vi "bats.parser.vi"(10 "niInstr IPv4 UDP Data Stream out":refnum<class "niInstr IPv4 UDP Data Stream v1.lvclass">, 11 "reset":bool) -> (2 "Ready.for.Udp.Input":bool)   [LabVIEW 2020]
uses:
  <instrlib>/_niInstr/Network/IPv4/UDP/Data Stream/v1/niInstr IPv4 UDP Data Stream v1.lvclass
  bats.parser.state.data.ctl
  bats.parser.state.command.ctl
  debug/debug.type.ctl
  <instrlib>/_niInstr/Network/IPv4/UDP/Data Stream/v1/Read Data Stream.vi
  <vilib>/rvi/Emulation/niFpgaEmulationIsFPGAContextNoSignature.vi
  <vilib>/rvi/Emulation/niFpgaSctlEmulationGetInTimedLoop.vi
  <vilib>/rvi/errors/niFpgaSetErrorForExecOnDevCompSimple.vi
  <vilib>/rvi/eio/common/nirviEmuReportErrorAndStop.vi
  <vilib>/rvi/DataTransferAndStorage/Container/Common/niFpgaContainerGetUniqueNameForEmu.vi
  <vilib>/rvi/FIFO/Fifo_Resource/nirvififoEmulationSetSize.vi
  <vilib>/rvi/FIFO/Fifo_Resource/nirviFifoEmulationQueueMgr.vi
  <instcachedir>/0/nirviFifoEmulationQueueMgr_E5CAEC123FF24DC58D834DCA3CDAA9B5.lvgen/nirviFifoEmulationQueueMgr_E5CAEC123FF24DC58D834DCA3CDAA9B5_008.vi
  <vilib>/rvi/FIFO/Fifo_Resource/nirvififoEmulationDetermineInputValidOut.vi
  <vilib>/rvi/FIFO/Fifo_Resource/nirvififoEmulationCreateLock.vi
  <vilib>/rvi/Emulation/niFpgaProcessEmulError.vi
  <vilib>/rvi/FIFO/Fifo_Resource/nirvififoEmulationObtainLock.vi
  <vilib>/rvi/FIFO/Fifo_Resource/nirvififoEmulationReleaseLock.vi
  <vilib>/rvi/occurrence/nirviWaitOnOccurrenceBase.vi
  <vilib>/rvi/errors/nirviReportUnexpectedCaseInternalError.vi
  <vilib>/rvi/errors/nirviReportUnexpectedCaseInternalError (U32).vi
  <instcachedir>/0/nirviFifoEmulationQueueMgr_E5CAEC123FF24DC58D834DCA3CDAA9B5.lvgen/nirviFifoEmulationQueueMgr_E5CAEC123FF24DC58D834DCA3CDAA9B5_006.vi
  <vilib>/rvi/DataTransferAndStorage/Container/XNode/niFpgaContainer.xnode
  <vilib>/rvi/FIFO/Fifo_Resource/nirvififoEmulationWrite.vi
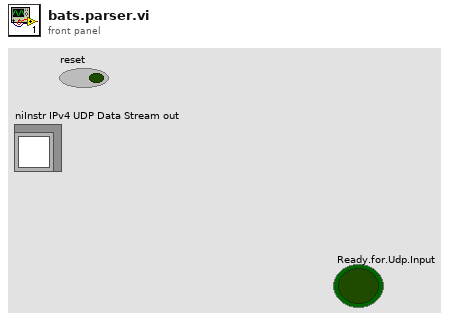
[diagram p1: front panel]
types:
  T1 = typedef "bats.parser.state.command.ctl" = enum16{"Reset", "Noop", "Read.Sequenced.Unit.Header", "Read.Msg"}
  T2 = typedef "bats.parser.state.data.ctl" = cluster{"BATS.Parser.States":T1, "Saved.BATS.Parser.State":T1, "Hdr Length (U16)":u16, "MessageLength (U8)":u8, "MessageType (U8)":u8, "Time (U32)":u32, "Total Counter (U16)":u16, "Message Counter (U8)":u8, "i":u16, "Number.of.Tickers":u16, "n":u16, "msg.counter":u8, "msg.length":u8, "buffer.start":u8, "buffer.length":u8, "buffer":u64[], "Debug":T3, "Next.Seq.No":u32}
  T3 = typedef "debug.type.ctl" = cluster{"Write.to.Debug":bool, "Data":u64}
  T4 = typedef "niInstr Ethernet Utilities FPGA v1.lvlib/Network Data Stream.ctl" = cluster{"data":u8[], "data valid":bool, "byte enables":bool[]}
  T5 = typedef "fpganow.common.fpga.lvlib/orderbook.command.ctl" = cluster{"type":T6, "side":u8, "orderId ":u64, "quantity":u32, "symbol":u64, "price":u64, "executed.qty":u32, "canceled.qty":u32, "remaining.qty":u32, "seconds":u64, "nanoseconds":u64, "Add":bool, "Edit":bool, "Remove":bool, "seq no":u32}
  T6 = typedef "fpganow.common.fpga.lvlib/orderbook.command.type.ctl" = enum8{"Time", "AddOrder", "OrderExecuted", "OrderExecutedAtPrice", "ReduceSize", "ModifyOrder", "DeleteOrder", "Get.Everything", "Get.All.Orders", "Get.Top"}
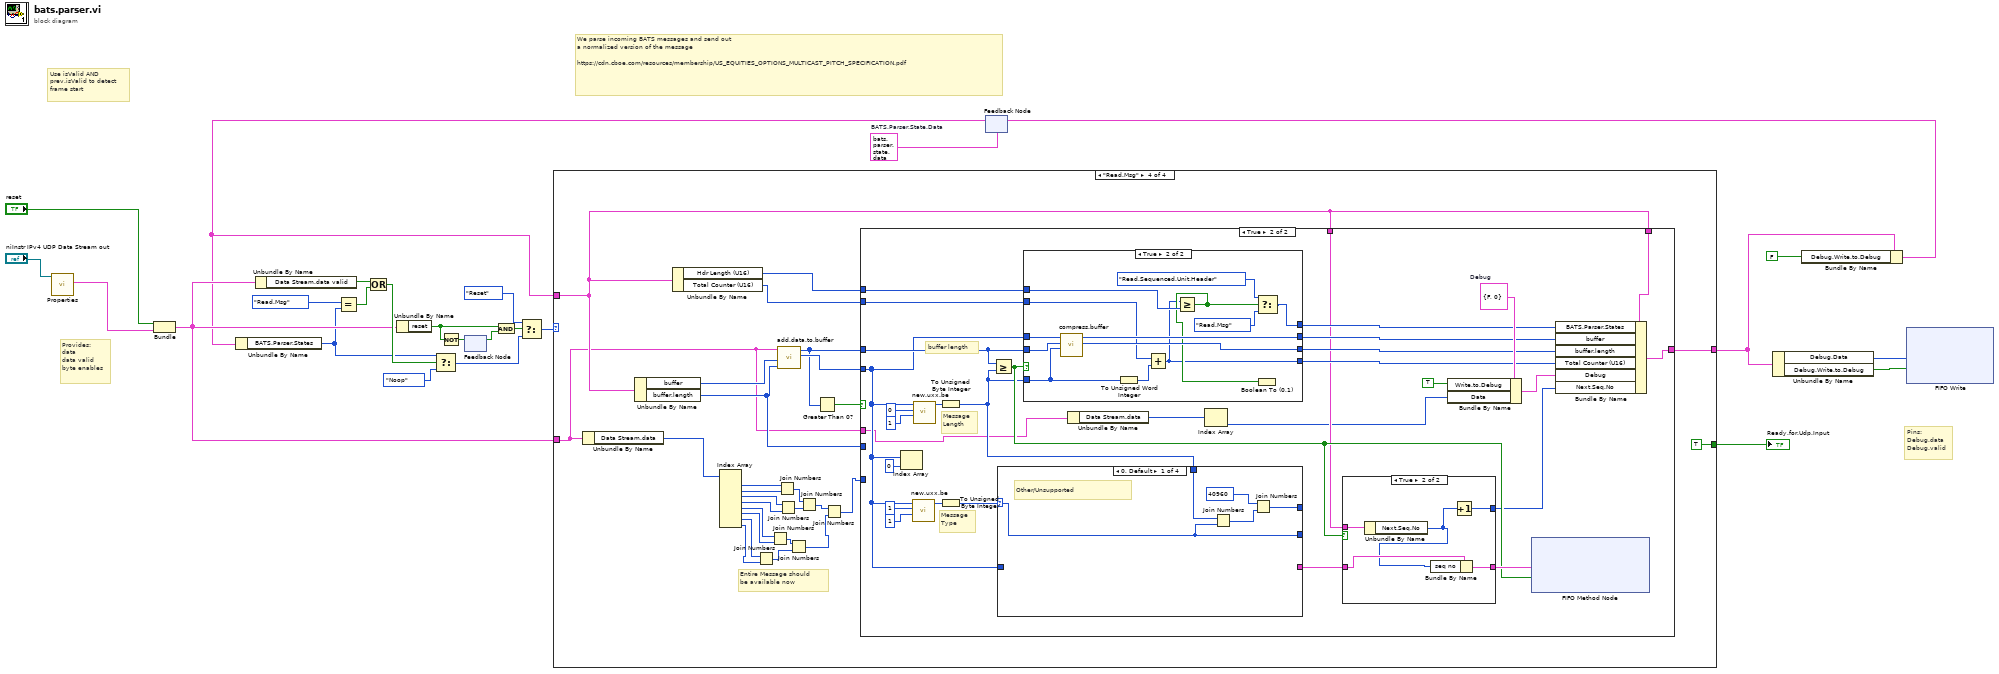
[diagram p0: block diagram]
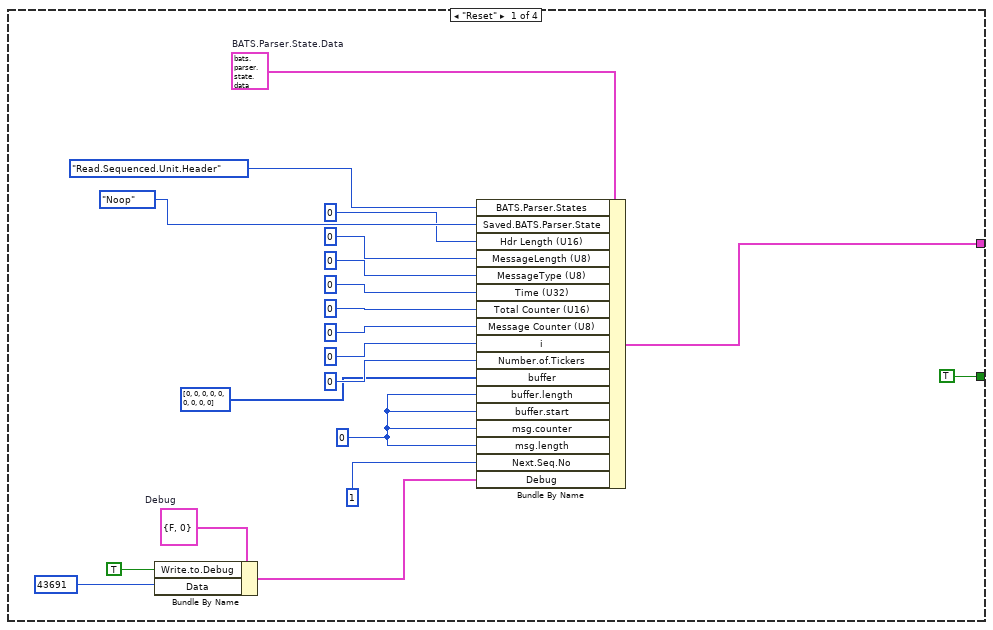
[diagram p2: hidden frame]
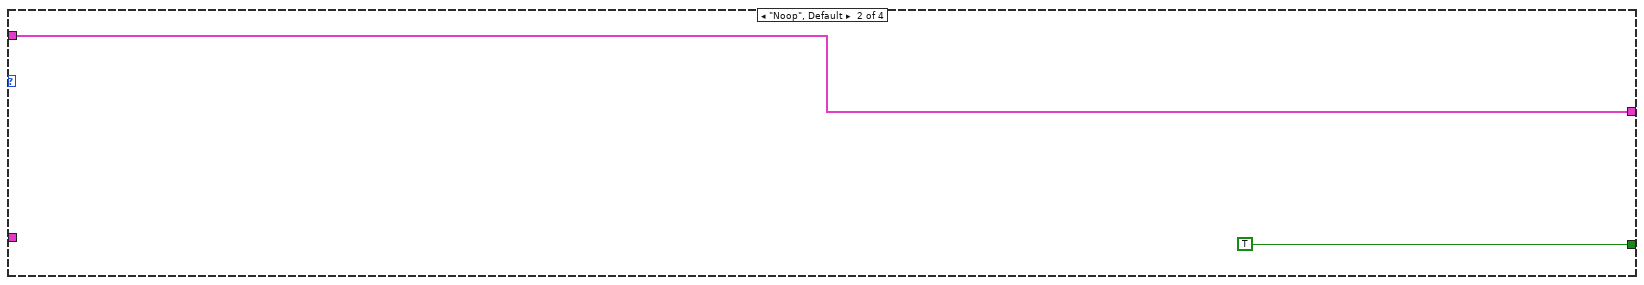
[diagram p3: hidden frame]
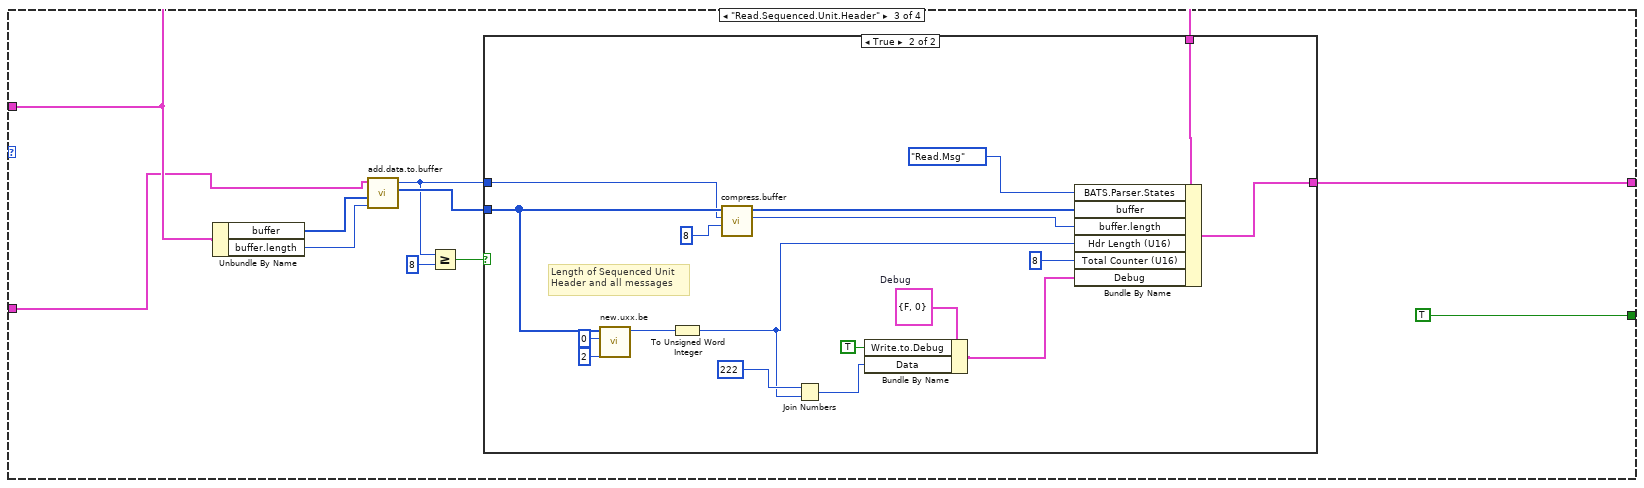
[diagram p4: hidden frame]
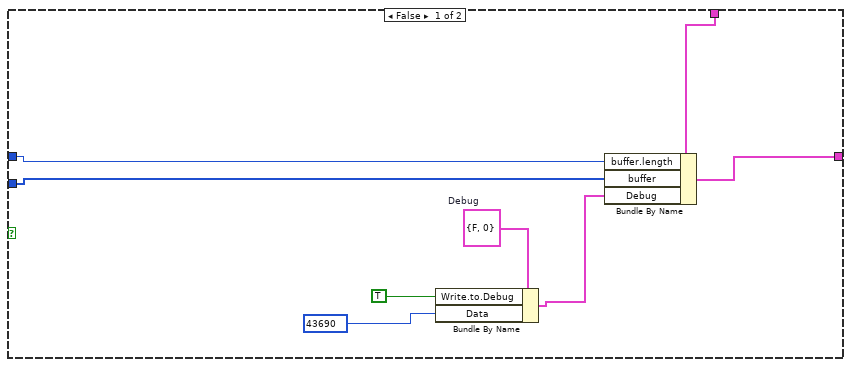
[diagram p5: hidden frame]
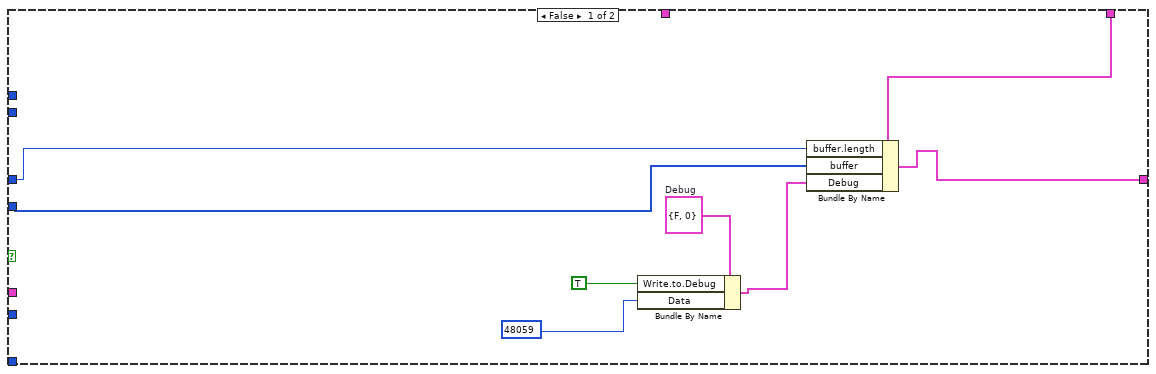
[diagram p6: hidden frame]
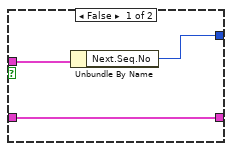
[diagram p7: hidden frame]
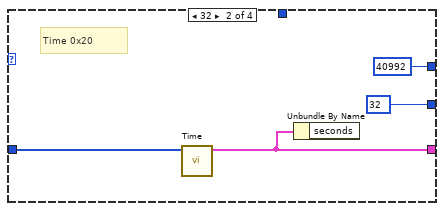
[diagram p8: hidden frame]
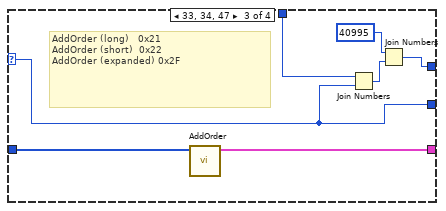
[diagram p9: hidden frame]
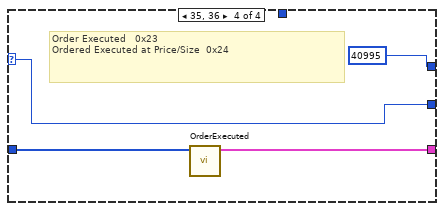
[diagram p10: hidden frame]
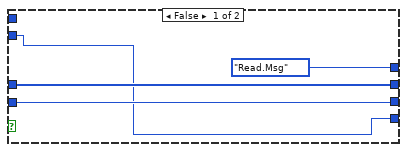
[diagram p11: hidden frame]
diagram:
  w25 = T2 {"BATS.Parser.States"=enum."Read.Sequenced.Unit.Header", "Saved.BATS.Parser.State"=enum."Reset", "Hdr Length (U16)"=0, "MessageLength (U8)"=0, "MessageType (U8)"=0, "Time (U32)"=0, "Total Counter (U16)"=0, "Message Counter (U8)"=0, "i"=0, "Number.of.Tickers"=0, "n"=0, "msg.counter"=0, "msg.length"=0, "buffer.start"=0, "buffer.length"=0, "buffer"=[0, 0, 0, 0, 0, 0, 0, 0, 0], "Debug"={"Write.to.Debug"=FALSE, "Data"=0}, "Next.Seq.No"=0}  # BATS.Parser.State.Data
  # "Use isValid AND\nprev.isValid to detect\nframe start"
  # "Provides:\ndata\ndata valid\nbyte enables"
  # "Pins:\nDebug.data\nDebug.valid"
  # "We parse incoming BATS messages and send out\na normalized version of the message\n\nhttps://cdn.cboe.com/resources/membership/US_EQUITIES_OPTIONS_MULTICAST_PITCH_SPECIFICATION.pdf"
  n1 = call-poly <instrlib>:"Properties.vi"("niInstr IPv4 UDP Data Stream v1.lvclass"="niInstr IPv4 UDP Data Stream out") -> ("Data Stream"=w2:T4)  [unwired: 9 in, 1 out]
  n2 = Bundle("reset"="reset", "Data Stream"=w2) -> (w9:cluster{"reset":bool, "Data Stream":T4})  [unwired: 1 in]
  n3 = Unbundle By Name(w9) -> ("Data Stream.data valid"=w12:bool)
  n4 = Unbundle By Name(w9) -> ("reset"=w15:bool)
  n5 = Not(x=w15) -> (.not. x?=w17:bool)
  n6 = feedback-in #1(w17) -> ()
  n7 = feedback #1() -> (w18:bool)  [unwired: 1 in]
  n8 = And(x=w15, y=w18) -> (x .and. y?=w19:bool)
  n9 = feedback #2(w25) -> (w1:T2)
  n10 = Unbundle By Name(w1) -> ("BATS.Parser.States"=w8:T1)
  n11 = Equal?(x=bats.parser.state.command."Read.Msg" ("BATS.Parser.States"), y=w8) -> (x = y?=w20:bool)
  n12 = Compound Arithmetic op=OR(w12, w20) -> (w11:bool)
  n13 = Select(t=w8, s=w11, f=bats.parser.state.command."Noop" ("BATS.Parser.States")) -> (s? t:f=w10:T1)
  n14 = Select(t=bats.parser.state.command."Reset" ("BATS.Parser.States"), s=w19, f=w10) -> (s? t:f=w22:T1)
  n15 = case shown="\"Read.Msg\"" w22 {
    tunnel: w1 -> [_ w47 w53 w102]
    tunnel: [w44 w47 w55 w110] -> w4
    tunnel: [TRUE ("Ready for Input") TRUE ("Ready for Input") TRUE ("Ready for Input") TRUE ("Ready for Input")] -> w16
    tunnel: w9 -> [_ _ w48 w84]
    frame "Reset" {
      w33 = T3 {"Write.to.Debug"=FALSE, "Data"=0}  # Debug
      w27 = u8 0 ("buffer.length")
      w45 = T2 {"BATS.Parser.States"=enum."Read.Sequenced.Unit.Header", "Saved.BATS.Parser.State"=enum."Reset", "Hdr Length (U16)"=0, "MessageLength (U8)"=0, "MessageType (U8)"=0, "Time (U32)"=0, "Total Counter (U16)"=0, "Message Counter (U8)"=0, "i"=0, "Number.of.Tickers"=0, "n"=0, "msg.counter"=0, "msg.length"=0, "buffer.start"=0, "buffer.length"=0, "buffer"=[0, 0, 0, 0, 0, 0, 0, 0, 0], "Debug"={"Write.to.Debug"=FALSE, "Data"=0}, "Next.Seq.No"=0}  # BATS.Parser.State.Data
      n16 = Bundle By Name(cluster=w33, "Write.to.Debug"=TRUE, "Data"=u64 43691) -> (w28:T3)
      n17 = Bundle By Name(cluster=w45, "BATS.Parser.States"=bats.parser.state.command."Read.Sequenced.Unit.Header", "Saved.BATS.Parser.State"=bats.parser.state.command."Noop" ("BATS.Parser.States"), "Hdr Length (U16)"=u16 0, "MessageLength (U8)"=u8 0, "MessageType (U8)"=u8 0, "Time (U32)"=u32 0, "Total Counter (U16)"=u16 0, "Message Counter (U8)"=u8 0, "i"=u16 0, "Number.of.Tickers"=u16 0, "buffer"=u64[] [0, 0, 0, 0, 0, 0, 0, 0, 0], "buffer.length"=w27, "buffer.start"=w27, "msg.counter"=w27, "msg.length"=w27, "Next.Seq.No"=u32 1, "Debug"=w28) -> (w44:T2)
    }
    frame "Noop", Default {
    }
    frame "Read.Sequenced.Unit.Header" {
      n18 = Unbundle By Name(w53) -> ("buffer"=w57:u64[], "buffer.length"=w56:u8)
      n19 = call "add.data.to.buffer.vi"("buffer.length"=w56, "buffer"=w57, "network Data Stream.ctl"=w48) -> ("buffer.out"=w54:u64[], "buffer.length.out"=w51:u8)  [unwired: 7 in]
      n20 = Greater Or Equal?(x=w51, y=u8 8) -> (x >= y?=w52:bool)
      n21 = case shown="True" w52 {
        tunnel: [w62 w83] -> w55
        tunnel: w54 -> [w59 w78]
        tunnel: w51 -> [w60 w70]
        tunnel: w53 -> [w61 w81]
        frame False {
          w63 = T3 {"Write.to.Debug"=FALSE, "Data"=0}  # Debug
          n22 = Bundle By Name(cluster=w63, "Write.to.Debug"=TRUE, "Data"=u64 43690) -> (w65:T3)
          n23 = Bundle By Name(cluster=w61, "buffer.length"=w60, "buffer"=w59, "Debug"=w65) -> (w62:T2)
        }
        frame True {
          w74 = T3 {"Write.to.Debug"=FALSE, "Data"=0}  # Debug
          # "Length of Sequenced Unit\nHeader and all messages"
          n24 = call "new.uxx.be.vi"("buffer (U64)"=w78, "Start.Idx"=u8 0, "Length"=u8 2) -> ("Uxx.be"=w75:u64)  [unwired: 7 in]
          n25 = To Unsigned Word Integer(number=w75) -> (unsigned 16bit integer=w66:u16)
          n26 = call "compress.buffer.vi"("start.idx"=u8 8, "buffer.length"=w70, "buffer"=w78) -> ("buffer.length.out"=w69:u8, "buffer.out"=w76:u64[])  [unwired: 7 in]
          n27 = Join Numbers(hi=u32 222 ("Data"), lo=w66) -> ((hi.lo)=w67:u64)
          n28 = Bundle By Name(cluster=w74, "Write.to.Debug"=TRUE, "Data"=w67) -> (w72:T3)
          n29 = Bundle By Name(cluster=w81, "BATS.Parser.States"=bats.parser.state.command."Read.Msg", "buffer"=w76, "buffer.length"=w69, "Hdr Length (U16)"=w66, "Total Counter (U16)"=u16 8, "Debug"=w72) -> (w83:T2)
        }
      }
    }
    frame "Read.Msg" {
      # "Entire Message should \nbe available now"
      n30 = Unbundle By Name(w84) -> ("Data Stream.data"=w85:u8[])
      n31 = Unbundle By Name(w102) -> ("buffer"=w101:u64[], "buffer.length"=w104:u8)
      n32 = Unbundle By Name(w102) -> ("Hdr Length (U16)"=w106:u16, "Total Counter (U16)"=w105:u16)
      n33 = Index Array(array=w85) -> (element #1=w100:u8, element #2=w99:u8, element #3=w98:u8, element #4=w97:u8, element #5=w96:u8, element #6=w95:u8, element #7=w94:u8, element #8=w93:u8)  [unwired: 8 in]
      n34 = Join Numbers(hi=w94, lo=w93) -> ((hi.lo)=w92:u16)
      n35 = Join Numbers(hi=w96, lo=w95) -> ((hi.lo)=w91:u16)
      n36 = Join Numbers(hi=w100, lo=w99) -> ((hi.lo)=w89:u16)
      n37 = Join Numbers(hi=w98, lo=w97) -> ((hi.lo)=w90:u16)
      n38 = call "add.data.to.buffer.vi"("buffer.length"=w104, "buffer"=w101, "network Data Stream.ctl"=w84) -> ("buffer.out"=w109:u64[], "buffer.length.out"=w108:u8)  [unwired: 7 in]
      n39 = Join Numbers(hi=w91, lo=w92) -> ((hi.lo)=w87:u32)
      n40 = Join Numbers(hi=w89, lo=w90) -> ((hi.lo)=w88:u32)
      n41 = Greater Than 0?(x=w108) -> (x > 0?=w107:bool)
      n42 = Join Numbers(hi=w88, lo=w87) -> ((hi.lo)=w86:u64)
      n43 = case shown="True" w107 {
        tunnel: [w117 w148] -> w110
        tunnel: w109 -> [w116 w122]
        tunnel: w108 -> [w112 w133]
        tunnel: w102 -> [w118 w147]
        tunnel: w106 -> [_ w136]
        tunnel: w105 -> [_ w135]
        tunnel: w104 -> [_ _]
        tunnel: w102 -> [_ w124]
        tunnel: w86 -> [_ _]
        tunnel: w84 -> [_ w121]
        frame False {
          w113 = T3 {"Write.to.Debug"=FALSE, "Data"=0}  # Debug
          n44 = Bundle By Name(cluster=w113, "Write.to.Debug"=TRUE, "Data"=u64 48059) -> (w115:T3)
          n45 = Bundle By Name(cluster=w118, "buffer.length"=w112, "buffer"=w116, "Debug"=w115) -> (w117:T2)
        }
        frame True {
          w143 = T3 {"Write.to.Debug"=FALSE, "Data"=0}  # Debug
          # "buffer length"
          # "Message\nType"
          # "Message\nLength"
          n46 = Index Array(array=w122, index=0) -> ()  [unwired: 1 out]
          n47 = call "new.uxx.be.vi"("buffer (U64)"=w122, "Start.Idx"=u8 1, "Length"=u8 1) -> ("Uxx.be"=w141:u64)  [unwired: 7 in]
          n48 = call "new.uxx.be.vi"("buffer (U64)"=w122, "Start.Idx"=u8 0, "Length"=u8 1) -> ("Uxx.be"=w144:u64)  [unwired: 7 in]
          n49 = To Unsigned Byte Integer(number=w144) -> (unsigned 8bit integer=w123:u8)
          n50 = To Unsigned Byte Integer(number=w141) -> (unsigned 8bit integer=w130:u8)
          n51 = Greater Or Equal?(x=w133, y=w123) -> (x >= y?=w126:bool)
          n52 = case shown="0, Default" w130 {
            selector: w130 -> [w158 _ w166 w174]
            tunnel: [w158 u64 32 ("unsigned 8bit integer") w166 w174] -> _
            tunnel: [_ w163 w172 w176] -> w128
            tunnel: w122 -> [_ w165 w171 w175]
            tunnel: [w160 u64 40992 ("seconds") w169 u64 40995 ("seconds")] -> _
            tunnel: w123 -> [w159 _ w168 _]
            frame 0, Default {
              # "Other/Unsupported"
              n53 = Join Numbers(hi=w159, lo=w158) -> ((hi.lo)=w157:u16)
              n54 = Join Numbers(hi=u64 40960 ("seconds"), lo=w157) -> ((hi.lo)=w160:u64)
            }
            frame 32 {
              # "Time 0x20"
              n55 = call "Time.vi"("buffer.in"=w165) -> ("OrderBook.Command"=w163:T5)  [unwired: 10 in]
              n56 = Unbundle By Name(w163) -> ()  [unwired: 1 out]
            }
            frame 33, 34, 47 {
              # "AddOrder (long)   0x21\nAddOrder (short)  0x22\nAddOrder (expanded) 0x2F"
              n57 = call "AddOrder.vi"("buffer.in"=w171) -> ("OrderBook.Command"=w172:T5)  [unwired: 10 in]
              n58 = Join Numbers(hi=w168, lo=w166) -> ((hi.lo)=w167:u16)
              n59 = Join Numbers(hi=u64 40995 ("seconds"), lo=w167) -> ((hi.lo)=w169:u64)
            }
            frame 35, 36 {
              # "Order Executed   0x23\nOrdered Executed at Price/Size  0x24"
              n60 = call "OrderExecuted.vi"("buffer.in"=w175) -> ("OrderBook.Command"=w176:T5)  [unwired: 10 in]
            }
          }
          n61 = case shown="True" w126 {
            tunnel: [w179 w190] -> w139
            tunnel: [w180 w193] -> w140
            tunnel: w133 -> [w179 w191]
            tunnel: w122 -> [w180 w192]
            tunnel: w123 -> [_ w189]
            tunnel: [bats.parser.state.command."Read.Msg" ("BATS.Parser.States") w184] -> w138
            tunnel: [w177 w181] -> w137
            tunnel: w136 -> [_ w186]
            tunnel: w135 -> [w177 w187]
            frame False {
            }
            frame True {
              n62 = call "compress.buffer.vi"("start.idx"=w189, "buffer.length"=w191, "buffer"=w192) -> ("buffer.length.out"=w190:u8, "buffer.out"=w193:u64[])  [unwired: 7 in]
              n63 = To Unsigned Word Integer(number=w189) -> (unsigned 16bit integer=w188:u16)
              n64 = Add(x=w187, y=w188) -> (x+y=w181:u16)
              n65 = Greater Or Equal?(x=w181, y=w186) -> (x >= y?=w182:bool)
              n66 = Boolean To (0,1)(Boolean=w182) -> ()  [unwired: 1 out]
              n67 = Select(t=bats.parser.state.command."Read.Sequenced.Unit.Header", s=w182, f=bats.parser.state.command."Read.Msg" ("BATS.Parser.States")) -> (s? t:f=w184:T1)
            }
          }
          n68 = Unbundle By Name(w121) -> ("Data Stream.data"=w120:u8[])
          n69 = Index Array(array=w120) -> (element=w119:u8)  [unwired: 1 in]
          n70 = case shown="True" w126 {
            tunnel: w128 -> [w151 w156]
            tunnel: [w151 w155] -> w127
            tunnel: w124 -> [w149 w154]
            tunnel: [w150 w152] -> w125
            frame False {
              n71 = Unbundle By Name(w149) -> ("Next.Seq.No"=w150:u32)
            }
            frame True {
              n72 = Unbundle By Name(w154) -> ("Next.Seq.No"=w153:u32)
              n73 = Bundle By Name(cluster=w156, "seq no"=w153) -> (w155:T5)
              n74 = Increment(x=w153) -> (x+1=w152:u32)
            }
          }
          n75 = Bundle By Name(cluster=w143, "Write.to.Debug"=TRUE, "Data"=w119) -> (w134:T3)
          n76 = xnode ("FIFO Method Node")("Element"=w127, "Input Valid"=w126) -> ()  [unwired: 1 in, 2 out]
          n77 = Bundle By Name(cluster=w147, "BATS.Parser.States"=w138, "buffer"=w140, "buffer.length"=w139, "Total Counter (U16)"=w137, "Debug"=w134, "Next.Seq.No"=w125) -> (w148:T2)
        }
      }
    }
  }
  "Ready.for.Udp.Input" <- w16
  n78 = Unbundle By Name(w4) -> ("Debug.Data"=w7:u64, "Debug.Write.to.Debug"=w5:bool)
  n79 = Bundle By Name(cluster=w4, "Debug.Write.to.Debug"=FALSE) -> (w14:T2)
  n80 = feedback-in #2(w14) -> ()
  n81 = xnode ("FIFO Write")("Element"=w7, "Input Valid"=w5) -> ()  [unwired: 1 in, 2 out]
